vi "Panther Dashboard for DQMH.vi"(8 "error in":errorcluster, 10 "Theme Dark=True":bool=TRUE, 11 "Include Dependencies (T)":bool=TRUE) -> (0 "error out":errorcluster)   [LabVIEW 2019]
uses:
  Panther Dashboard/Panther Dashboard.lvlib
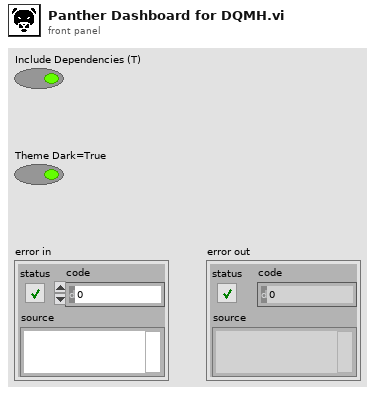
[diagram p1: front panel]
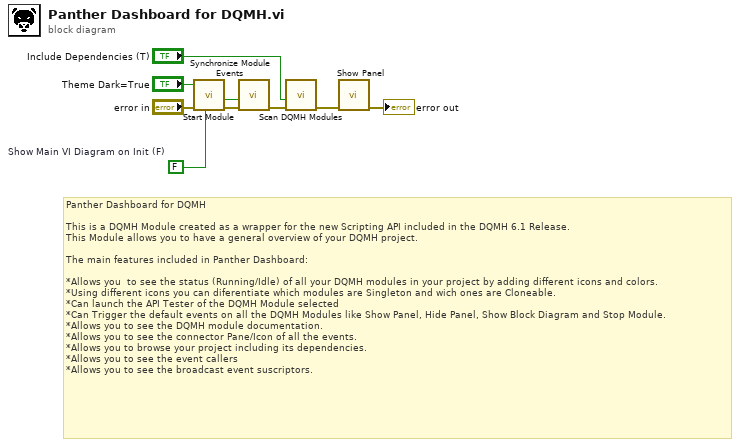
[diagram p0: block diagram]
diagram:
  w2 = FALSE  # Show Main VI Diagram on Init (F)
  # "Panther Dashboard for DQMH\n\nThis is a DQMH Module created as a wrapper for the new Scripting API included in the DQMH 6.1 Release.\nThis Module allows you to have a general overview of your DQMH project.\n\nThe main features included in Panther Dashboard:\n\n*Allows you  to see the status (Running/Idle) of all your DQMH modules in your project by adding different icons and colors.\n*Using different icons you can diferentiate which modules are Singleton and wich ones are Cloneable.\n*Can launch the API Tester of the DQMH Module selected\n*Can Trigger the default events on all the DQMH Modules like Show Panel, Hide Panel, Show Block Diagram and Stop Module.\n*Allows you to see the DQMH module documentation.\n*Allows you to see the connector Pane/Icon of all the events.\n*Allows you to browse your project including its dependencies.\n*Allows you to see the event callers\n*Allows you to see the broadcast event suscriptors."
  n1 = call "Start Module.vi"("Show Main VI Diagram on Init (F)"=w2, "error in"="error in", "Theme Dark=True"="Theme Dark=True") -> ("error out"=w9:errorcluster, "Wait for Event Sync?"=w4:bool)  [unwired: 5 in, 2 out]
  n2 = call "Synchronize Module Events.vi"("error in"=w9, "Wait for Event Sync?"=w4) -> ("error out"=w8:errorcluster)  [unwired: 9 in]
  n3 = call "Scan DQMH Modules.vi"("error in"=w8, "Include Dependencies"="Include Dependencies (T)") -> ("error out"=w7:errorcluster)  [unwired: 9 in]
  n4 = call "Show Panel.vi"("error in (no error)"=w7) -> ("error out"=→"error out":errorcluster)  [unwired: 10 in]
